vi "Safe Hardware.vi"(8 "error in (no error)":errorcluster, 11 "Process Settings in":refnum<class "Process Settings.lvclass">) -> (0 "error out":errorcluster, 3 "Process Settings out":refnum<class "Process Settings.lvclass">)   [LabVIEW 2017, in "Expansion.lvclass"]
uses:
  Expansion.lvclass
  Process Settings/Process Settings.lvclass
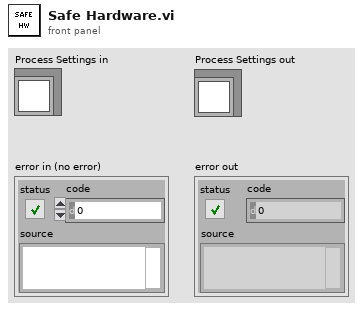
[diagram p1: front panel]
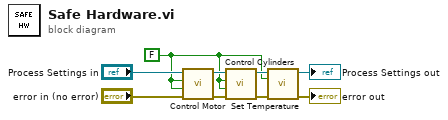
[diagram p0: block diagram]
diagram:
  w1 = FALSE ("Motor Power")
  n1 = call "Control Motor.vi"("error in (no error)"="error in (no error)", "Motor Power"=w1, "Motor Direction"=w1, "Process Settings in"="Process Settings in") -> ("error out"=w4:errorcluster, "Process Settings out"=w2:refnum<class "Process Settings.lvclass">)  [unwired: 6 in]
  n2 = call "Control Cylinders.vi"("error in (no error)"=w4, "Cylinder 2"=w1, "Cylinder 1"=w1, "Process Settings in"=w2) -> ("error out"=w5:errorcluster, "Process Settings out"=w9:refnum<class "Process Settings.lvclass">)  [unwired: 6 in]
  n3 = call "Set Temperature.vi"("error in (no error)"=w5, "On/Off"=w1, "Process Settings in"=w9) -> ("error out"=→"error out":errorcluster, "Process Settings out"=→"Process Settings out":refnum<class "Process Settings.lvclass">)  [unwired: 7 in]
